vi "NTC_R2T.vi"(11 "Resistance":dbl) -> (3 "Temperature":dbl)   [LabVIEW 2014]
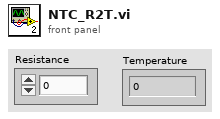
[diagram p1: front panel]
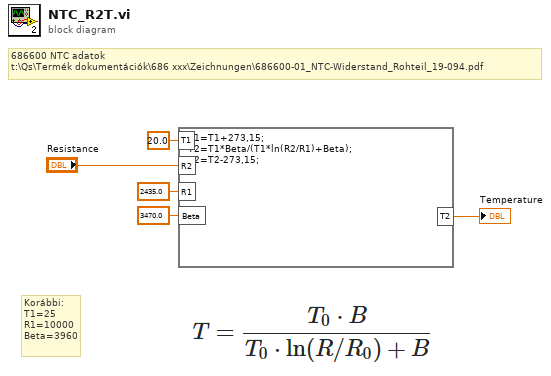
[diagram p0: block diagram]
diagram:
  # "686600 NTC adatok\nt:\\Qs\\Termék dokumentációk\\686 xxx\\Zeichnungen\\686600-01_NTC-Widerstand_Rohteil_19-094.pdf"
  # "Korábbi:\nT1=25\nR1=10000\nBeta=3960"
  n1 = formula code="T1=T1+273,15;\nT2=T1*Beta/(T1*ln(R2/R1)+Beta);\nT2=T2-273,15;"("T1"=20.0 ("input variable"), "R2"="Resistance", "R1"=2435.0 ("input variable"), "Beta"=3470.0 ("input variable")) -> ("T2"=→"Temperature":dbl)
